vi "Test Torque Calculations.vi"() -> ()   [LabVIEW 2016]
uses:
  Desktop/05-28/RT/Pedals Status.ctl
panel:
  in  "Velocity actual value":i32
  in  "\"Pedals\" Status":T1 {"Acceleration pedal" scale=0.0..100.0 scale format="%#_6f%%"; "Break pedal" scale=0.0..100.0 scale format="%#_6f%%"}
  out "Target Torque Left":i16(knob) scale=-666.0..666.0
  out "Target Torque Right":i16(knob) scale=666.0..-666.0
  out "Error Out":errorcluster
  in  "Error In":errorcluster
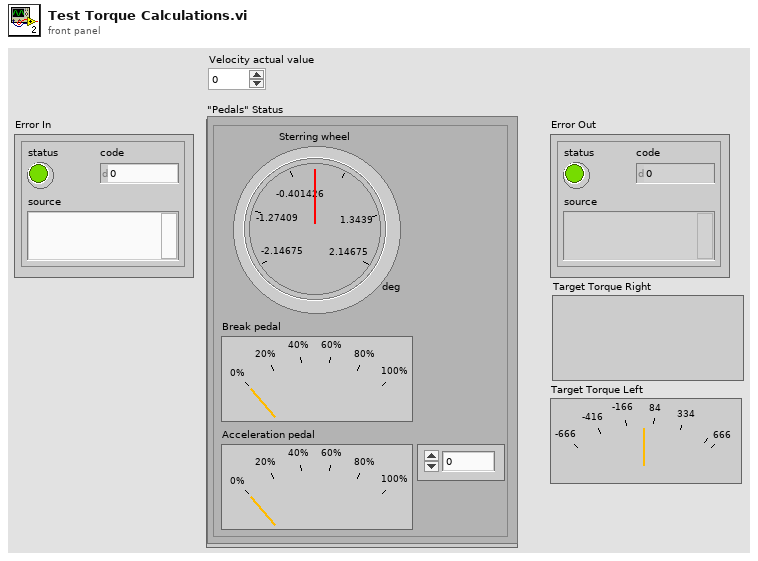
[diagram p1: front panel]
types:
  T1 = typedef "Pedals Status.ctl" = cluster{"Acceleration pedal":dbl, "Break pedal":dbl, "Sterring wheel":dbl[unit]}
  T2 = cluster{"Statusword":u16, "Warnings":u16, "Error code":u16, "Error register":u8, "Controller temperature":u8, "Motor temperature":u8, "Troque actual value":i16, "Velocity actual value":i32, "Electric power":u32, "DC current":u32, "Phase A current":u16, "Phase B current":u16, "Electrical Angle":u16}
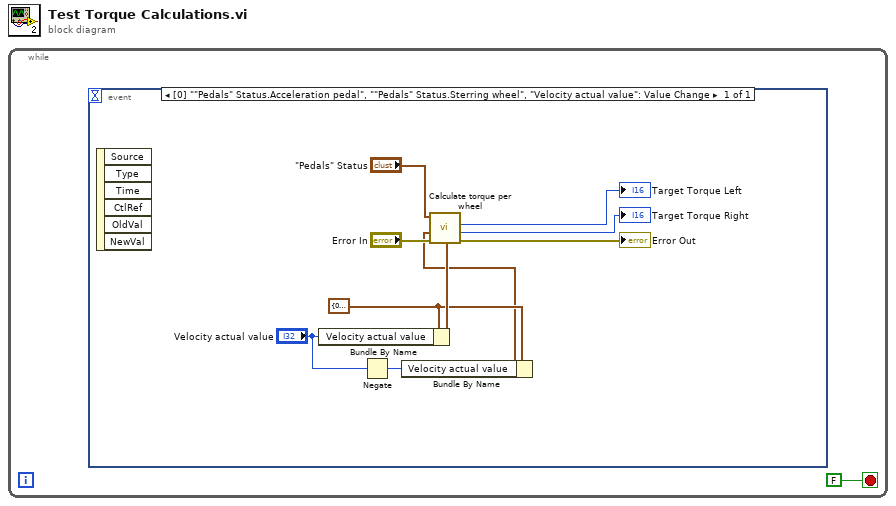
[diagram p0: block diagram]
diagram:
  n1 = while {
    stop <- FALSE stop-if-true
    n2 = event shown="[0] \"\"Pedals\" Status.Acceleration pedal\", \"\"Pedals\" Status.Sterring wheel\", \"Velocity actual value\": Value Change" {
      selector: _ -> [_]
      dyn-events: _ -> [_]
      timeout: _ -> [_]
      event "Velocity actual value": Value Change {
        w5 = T2 {"Statusword"=0, "Warnings"=0, "Error code"=0, "Error register"=0, "Controller temperature"=0, "Motor temperature"=0, "Troque actual value"=0, "Velocity actual value"=0, "Electric power"=0, "DC current"=0, "Phase A current"=0, "Phase B current"=0, "Electrical Angle"=0} ("Left Motor Status")
        n3 = event-data() -> ()  [unwired: 1 in, 6 out]
        n4 = Bundle By Name(cluster=w5, "Velocity actual value"="Velocity actual value") -> (w6:T2)
        n5 = Negate(x="Velocity actual value") -> (-x=w3:i32)
        n6 = Bundle By Name(cluster=w5, "Velocity actual value"=w3) -> (w4:T2)
        n7 = call "Calculate torque per wheel.vi"("Error In"="Error In", "Right Motor Status"=w4, "Left Motor Status"=w6, "\"Pedals\" Status"="\"Pedals\" Status") -> ("Error Out"=→"Error Out":errorcluster, "Target Torque Right"=→"Target Torque Right":i16, "Target Torque Left"=→"Target Torque Left":i16)  [unwired: 5 in]
      }
    }
  }
